vi "ConfigDlg.vi"(8 "error in (no error)":errorcluster, 11 "PMUAnalysis in":refnum<class "PmuAnalysis.lvclass">) -> (0 "error out":errorcluster, 2 "Changed":bool, 3 "PMUAnalysis out":refnum<class "PmuAnalysis.lvclass">)   [LabVIEW 2014, in "AnalysisPlugins.lvlib" / "PmuAnalysis.lvclass"]
uses:
  PmuAnalysis.lvclass
  FitterBaseClass/Typedefs/clAnalysisConfig.ctl
  AnalysisPluginBaseClass/AnalysisPluginsBase.lvclass/AnalysisPluginsBase.ctl
  PmuAnalysis.lvclass/PmuAnalysis.ctl
  <userlib>/NIST/BaseClasses/BasePlugin_class/BasePlugin.lvclass/BasePlugin.ctl
  <userlib>/NIST/BaseClasses/BasePlugin_class/Accessors/Read PluginIniFilePath.vi
  Accessors/Write eTestType.vi
  Accessors/Write FunctionIniFilePath.vi
  Accessors/Read Function.vi
  Accessors/Write Function.vi
  AnalysisPluginBaseClass/Accessors/Read DelayCorr.vi
  AnalysisPluginBaseClass/Accessors/Read MagCorr.vi
  Accessors/Read eTestType.vi
  Accessors/Read FunctionIniFilePath.vi
  FGen/MemberClasses/FunctionBaseClass/FunctionBase.lvclass
  <vilib>/Utility/config.llb/NI_LVConfig.lvlib
  FitterBaseClass/FitterBase.lvclass
panel:
  in  "btnFuncConfig":bool
  in  "FunctionIniFilePath":path caption="Test Function .ini File"
  in  "eTestType":T1(ring) caption="Test Type"
  in  "clAnalysisConfig":T2
  in  "BtnCancel":bool
  in  "MagCorr":dbl[](array[numeric])
  in  "DelayCorr":dbl[](array[numeric])
  in  "btnDone":bool
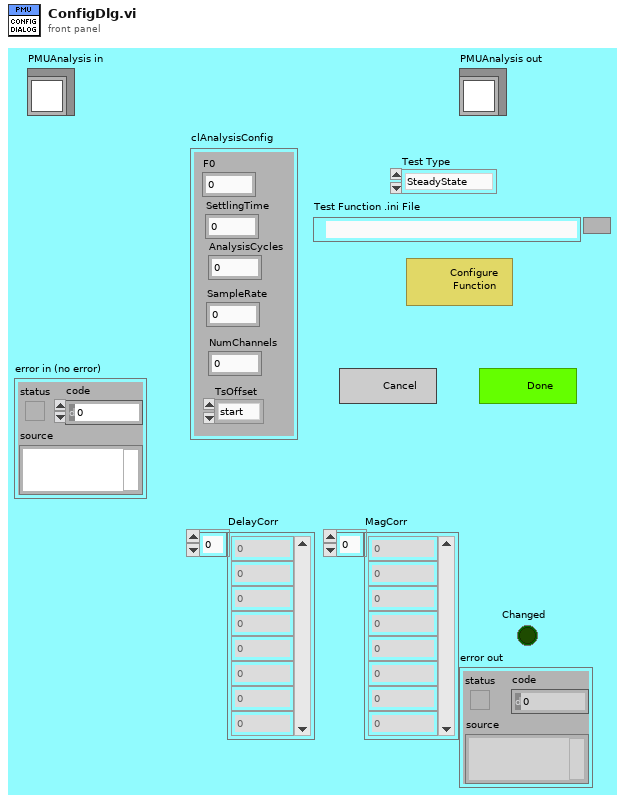
[diagram p1: front panel]
types:
  T1 = enum16{"SteadyState", "Modulation", "Ramp", "Step"}
  T2 = typedef "AnalysisPlugins.lvlib/FitterBase.lvclass/clAnalysisConfig.ctl" = cluster{"F0":u32, "SettlingTime":dbl, "AnalysisCycles":dbl, "SampleRate":dbl, "NumChannels":u32, "TsOffset":enum16{"start", "middle", "end"}}
  T3 = enum32{"Invalid", "Standard", "Closed", "Hidden", "Minimized", "Maximized"}
  T4 = enum32{"Invalid", "Default", "Floating", "Floating/Auto-Hide", "Modal"}
  T5 = typedef "AnalysisPlugins.lvlib/PmuAnalysis.lvclass/clAnalysisConfig.ctl" = cluster{"F0":u32, "SettlingTime":dbl, "AnalysisCycles":dbl, "SampleRate":dbl, "NumChannels":u32, "TsOffset":enum16{"start", "middle", "end"}}
  T6 = typedef "NI_LVConfig.lvlib/Config Data RefNum.ctl" = refnum<k1>
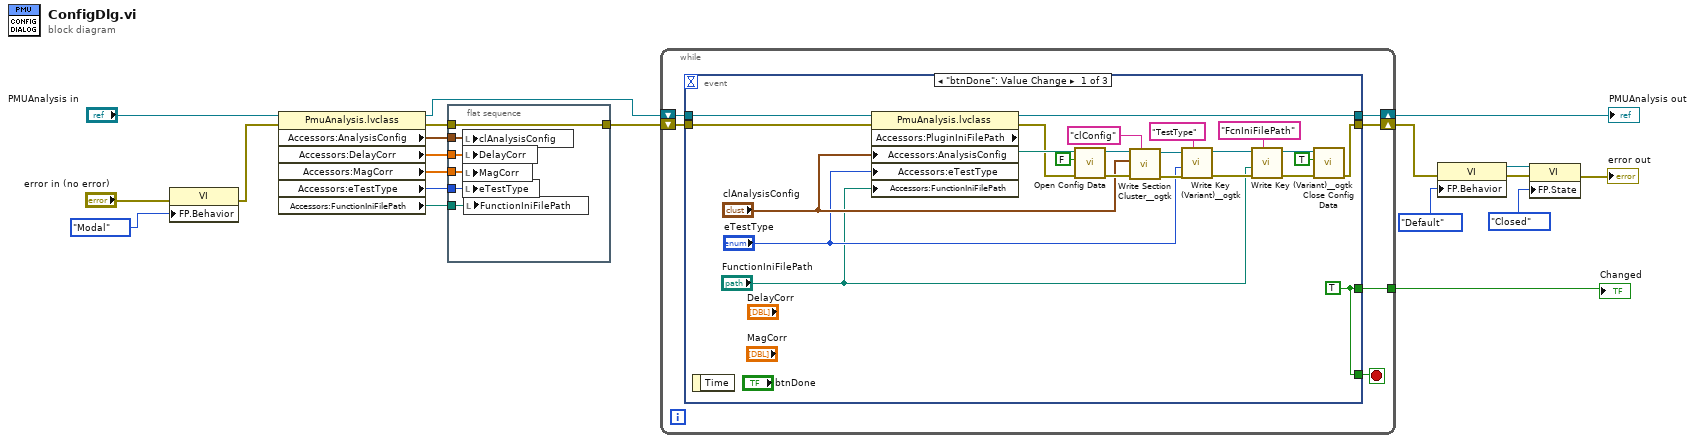
[diagram p0: block diagram]
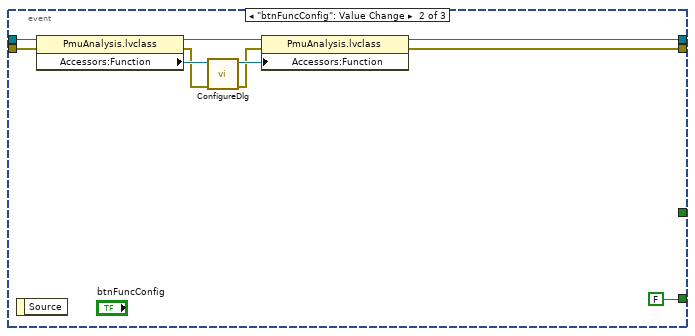
[diagram p2: hidden frame]
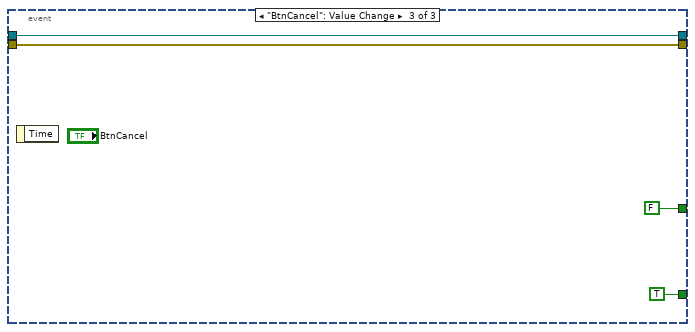
[diagram p3: hidden frame]
diagram:
  n1 = property class="VI"(error in="error in (no error)", "FP.Behavior"=T4."Modal" ("Front Panel Window:Behavior")) -> (error out=w14:errorcluster)  [unwired: 1 in, 1 out]
  n2 = property class="PmuAnalysis.lvclass"(reference="PMUAnalysis in", error in=w14) -> (reference out=w17:refnum<class "PmuAnalysis.lvclass">, error out=w6:errorcluster, "Accessors:AnalysisConfig"=w5:T5, "Accessors:DelayCorr"=w4:dbl[], "Accessors:MagCorr"=w3:dbl[], "Accessors:eTestType"=w7:T1, "Accessors:FunctionIniFilePath"=w1:path)
  n3 = flat-sequence {
    tunnel: w7 -> [w26]
    tunnel: w6 -> [w25]
    tunnel: [w25] -> w2
    tunnel: w5 -> [w24]
    tunnel: w4 -> [w23]
    tunnel: w3 -> [w22]
    tunnel: w1 -> [w21]
    frame #0 {
      n4 = local write "clAnalysisConfig"(w24) -> ()
      n5 = local write "DelayCorr"(w23) -> ()
      n6 = local write "MagCorr"(w22) -> ()
      n7 = local write "eTestType"(w26) -> ()
      n8 = local write "FunctionIniFilePath"(w21) -> ()
    }
  }
  n9 = while {
    tunnel: [w31] -> w18
    shift-right: [w32] -> w19
    shift-left: w17 -> [w30]
    shift-right: [w29] -> w13
    shift-left: w2 -> [w28]
    stop <- w27 stop-if-true
    n10 = event shown="[0] \"btnDone\": Value Change" {
      selector: _ -> [_ _ _]
      dyn-events: _ -> [_ _ _]
      timeout: _ -> [_ _ _]
      tunnel: [w46 w58 w69] -> w32
      tunnel: w30 -> [w55 w65 w69]
      tunnel: [w47 w57 w67] -> w29
      tunnel: [w33 _ FALSE] -> w31
      tunnel: w28 -> [w40 w64 w67]
      tunnel: [w33 FALSE TRUE] -> w27
      event "btnDone": Value Change {
        w33 = TRUE
        n11 = event-data() -> ()  [unwired: 1 in, 1 out]
        n12 = property class="PmuAnalysis.lvclass"(reference=w55, error in=w40, "Accessors:AnalysisConfig"="clAnalysisConfig", "Accessors:eTestType"="eTestType", "Accessors:FunctionIniFilePath"="FunctionIniFilePath") -> (reference out=w46:refnum<class "PmuAnalysis.lvclass">, error out=w52:errorcluster, "Accessors:PluginIniFilePath"=w54:path)
        n13 = call <vilib>:"Open Config Data.vi"("error in (no error)"=w52, "create file if necessary (T)"=FALSE, "configuration file path"=w54) -> ("error out"=w50:errorcluster, "refnum"=w49:T6)  [unwired: 6 in, 1 out]
        n14 = call <userlib>:"Write Section Cluster__ogtk.vi"("section (optional)"="clConfig", "error in (no error)"=w50, "Section Formatted Cluster"="clAnalysisConfig", "refnum"=w49) -> ("error out"=w44:errorcluster, "dup refnum"=w43:T6)  [unwired: 6 in]
        n15 = call <userlib>:"Write Key (Variant)__ogtk.vi"("section"="TestType", "error in (no error)"=w44, "key-value"="eTestType", "refnum"=w43) -> ("error out"=w39:errorcluster, "refnum out"=w38:T6)  [unwired: 6 in]
        n16 = call <userlib>:"Write Key (Variant)__ogtk.vi"("section"="FcnIniFilePath", "error in (no error)"=w39, "key-value"="FunctionIniFilePath", "refnum"=w38) -> ("error out"=w37:errorcluster, "refnum out"=w36:T6)  [unwired: 6 in]
        n17 = call <vilib>:"Close Config Data.vi"("error in (no error)"=w37, "write file if changed (T)"=TRUE, "refnum"=w36) -> ("error out"=w47:errorcluster)  [unwired: 7 in, 1 out]
      }
      event "btnFuncConfig": Value Change {
        n18 = event-data() -> ()  [unwired: 1 in, 1 out]
        n19 = property class="PmuAnalysis.lvclass"(reference=w65, error in=w64) -> (reference out=w61:refnum<class "PmuAnalysis.lvclass">, error out=w62:errorcluster, "Accessors:Function"=w63:refnum<class "FunctionBase.lvclass">)
        n20 = call-dynamic "ConfigureDlg.vi"("error in (no error)"=w62, "FunctionBase in"=w63) -> ("error out"=w59:errorcluster, "FunctionBase out"=w60:refnum<class "FunctionBase.lvclass">)  [unwired: 7 in, 1 out]
        n21 = property class="PmuAnalysis.lvclass"(reference=w61, error in=w59, "Accessors:Function"=w60) -> (reference out=w58:refnum<class "PmuAnalysis.lvclass">, error out=w57:errorcluster)
      }
      event "BtnCancel": Value Change {
        n22 = event-data() -> ()  [unwired: 1 in, 1 out]
      }
    }
  }
  "PMUAnalysis out" <- w19
  "Changed" <- w18
  n23 = property class="VI"(error in=w13, "FP.Behavior"=T4."Default" ("Front Panel Window:Behavior")) -> (reference out=w11:refnum<vi>, error out=w10:errorcluster)  [unwired: 1 in]
  n24 = property class="VI"(reference=w11, error in=w10, "FP.State"=T3."Closed" ("Front Panel Window:State")) -> (error out=→"error out":errorcluster)  [unwired: 1 out]
